vi "DAQ.Simulate Waveguide.vi"(8 "error in (no error)":errorcluster, 9 "Waveguide Cluster":T1={"Vsource Index"=0, "Vsg Index"=1, "V+"=0, "V-"=0}, 10 "AO []":waveform(dbl)[](array[waveform]), 11 "Instrument.DAQ in":refnum<class "Instrument.DAQ.lvclass">) -> (0 "error out":errorcluster, 2 "AI []":waveform(dbl)[](array[waveform]), 3 "Instrument.DAQ out":refnum<class "Instrument.DAQ.lvclass">)   [LabVIEW 2019, in "Instrument.Lockin.lvlib" / "Instrument.DAQ.lvclass"]
uses:
  Instrument.DAQ.lvclass
  Waveguide Model/Waveguide Model--Cluster.ctl
  Instrument.DAQ.lvclass/Instrument.DAQ.ctl
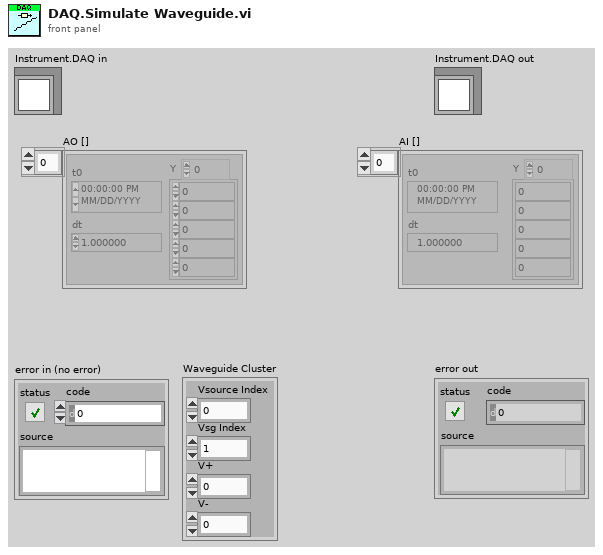
[diagram p1: front panel]
types:
  T1 = typedef "Instrument.Lockin.lvlib/Instrument.DAQ.lvclass/Waveguide Model--Cluster.ctl" = cluster{"Vsource Index":i32, "Vsg Index":i32, "V+":i32, "V-":i32}
  T2 = typedef "Instrument.Lockin.lvlib/Instrument.DAQ.lvclass/Channel.Gain--Cluster--Array.ctl" = T3[]
  T3 = typedef "Instrument.Lockin.lvlib/Instrument.DAQ.lvclass/Channel.Gain--Cluster.ctl" = cluster{"Channel":string, "Gain":dbl}
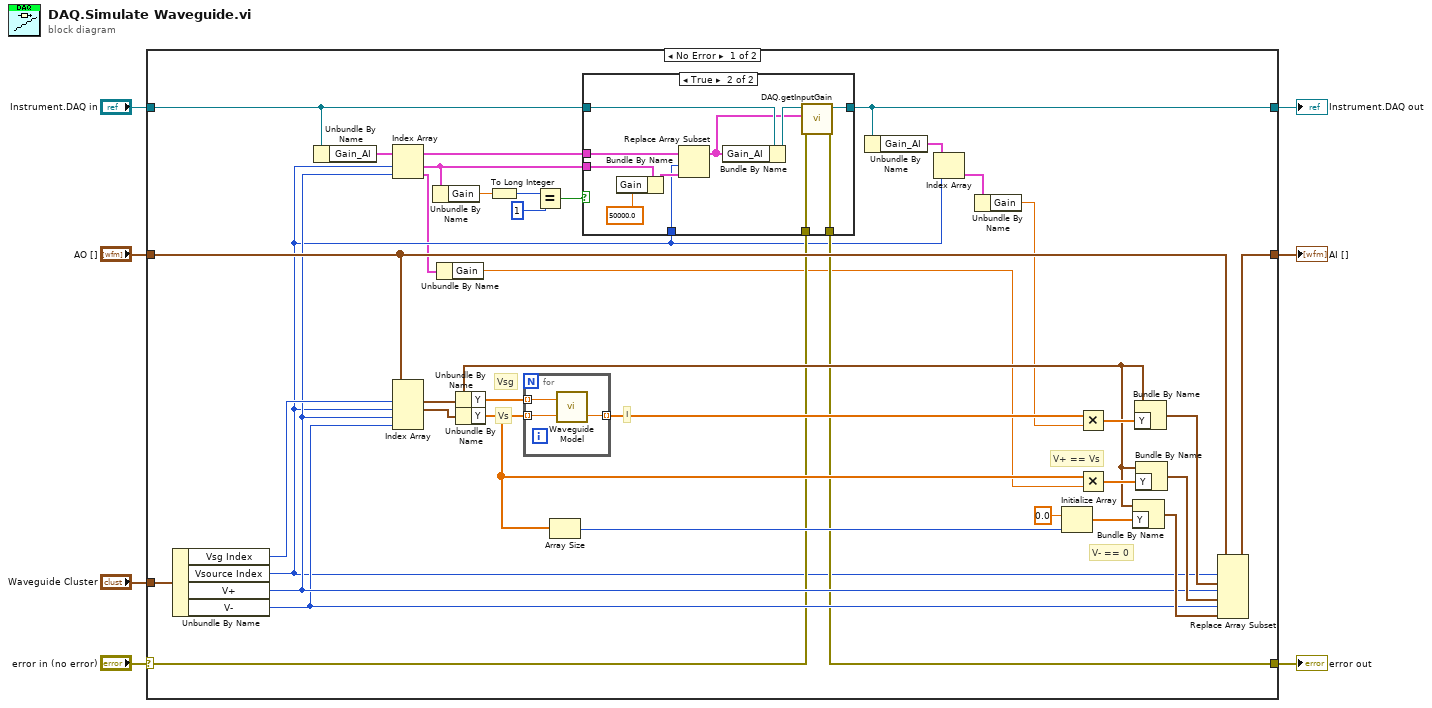
[diagram p0: block diagram]
diagram:
  n1 = case shown="No Error" "error in (no error)" {
    selector: "error in (no error)" -> [w12 w59]
    tunnel: "Waveguide Cluster" -> [w40 _]
    tunnel: [w37 w60] -> w6
    tunnel: [w11 w59] -> w4
    tunnel: [w16 w61] -> w3
    tunnel: "Instrument.DAQ in" -> [w17 w61]
    tunnel: "AO []" -> [w38 w60]
    frame No Error {
      # "V- == 0"
      # "V+ == Vs"
      # "I"
      # "Vs"
      # "Vsg"
      n2 = Unbundle By Name(w40) -> ("Vsg Index"=w36:i32, "Vsource Index"=w10:i32, "V+"=w24:i32, "V-"=w23:i32)
      n3 = Unbundle By Name(w17) -> ("Gain_AI"=w21:T2)
      n4 = Index Array(array=w21, index #1=w10, index #2=w24) -> (element #1=w20:T3, element #2=w9:T3)
      n5 = Index Array(array=w38, index #1=w36, index #2=w10, index #3=w24, index #4=w23) -> (element #1=w27:waveform(dbl), element #2=w35:waveform(dbl))  [unwired: 2 out]
      n6 = Unbundle By Name(w20) -> ("Gain"=w25:dbl)
      n7 = Unbundle By Name(w9) -> ("Gain"=w8:dbl)
      n8 = Unbundle By Name(w27) -> ("Y"=w39:dbl[])
      n9 = Unbundle By Name(w35) -> ("Y"=w31:dbl[])
      n10 = To Long Integer(number=w25) -> (32bit integer=w19:i32)
      n11 = for {
        tunnel: w31 -> [w58] mode=indexing
        tunnel: w39 -> [w57] mode=indexing
        tunnel: [w56] -> w42 mode=indexing
        n12 = call "Waveguide Model.vi"("Vs (V)"=w58, "Vsg (V)"=w57) -> ("I[Vsg] (A)"=w56:dbl)  [unwired: 1 out]
      }
      n13 = Equal?(x=w19, y=1 ("x")) -> (x = y?=w22:bool)
      n14 = Array Size(array=w31) -> (size(s)=w30:i32)
      n15 = case shown="True" w22 {
        tunnel: w21 -> [_ w55]
        tunnel: w20 -> [_ w54]
        tunnel: w10 -> [_ w48]
        tunnel: w17 -> [w44 w46]
        tunnel: [w44 w52] -> w16
        tunnel: w12 -> [w43 w50]
        tunnel: [w43 w49] -> w11
        frame False {
        }
        frame True {
          n16 = Bundle By Name(cluster=w54, "Gain"=50000.0) -> (w51:T3)
          n17 = Replace Array Subset(array=w55, new element=w51, index=w48) -> (w45:T2)
          n18 = Bundle By Name(cluster=w46, "Gain_AI"=w45) -> (w47:refnum<class "Instrument.DAQ.lvclass">)
          n19 = call "DAQ.getInputGain.vi"("error in (no error)"=w50, "Input Gain"=w45, "Instrument.DAQ"=w47) -> ("error out"=w49:errorcluster, "Instrument.DAQ out"=w52:refnum<class "Instrument.DAQ.lvclass">)  [unwired: 7 in]
        }
      }
      n20 = Unbundle By Name(w16) -> ("Gain_AI"=w15:T2)
      n21 = Index Array(array=w15, index=w10) -> (element=w14:T3)
      n22 = Unbundle By Name(w14) -> ("Gain"=w13:dbl)
      n23 = Initialize Array(0.0 ("y"), w30) -> (w28:dbl[])
      n24 = Multiply(x=w42, y=w13) -> (x*y=w41:dbl[])
      n25 = Multiply(x=w31, y=w8) -> (x*y=w33:dbl[])
      n26 = Bundle By Name(cluster=w27, "Y"=w28) -> (w26:waveform(dbl))
      n27 = Bundle By Name(cluster=w27, "Y"=w41) -> (w34:waveform(dbl))
      n28 = Bundle By Name(cluster=w27, "Y"=w33) -> (w32:waveform(dbl))
      n29 = Replace Array Subset(array=w38, new element #1=w34, index #1=w10, new element #2=w32, index #2=w24, new element #3=w26, index #3=w23) -> (w37:waveform(dbl)[])
    }
    frame Error {
    }
  }
  "error out" <- w4
  "Instrument.DAQ out" <- w3
  "AI []" <- w6
